vi "Get configuration chain.vi"(8 "error in (no error)":errorcluster, 11 "TemplateBase in":refnum<class "Cobolt.lvclass">) -> (0 "error out":errorcluster, 1 "class name":string[](array[string]), 2 "configuration chain":variant[](array[variant]), 3 "TemplateBase out":refnum<class "Cobolt.lvclass">)   [LabVIEW 2012, in "Cobolt.lvclass"]
doc: "Returns an array of variants containing the configuration clusters of each class in the inheritance chain (lowest child class first), together with an array of all class names in the inheritance chain.\n\nFor classes without configuration cluster, the configuration chain contains empty variants."
uses:
  Cobolt.lvclass
  <vilib>/Distrio/Murmex/Murmex/Murmex.lvclass
  Cobolt.lvclass/Cobolt.ctl
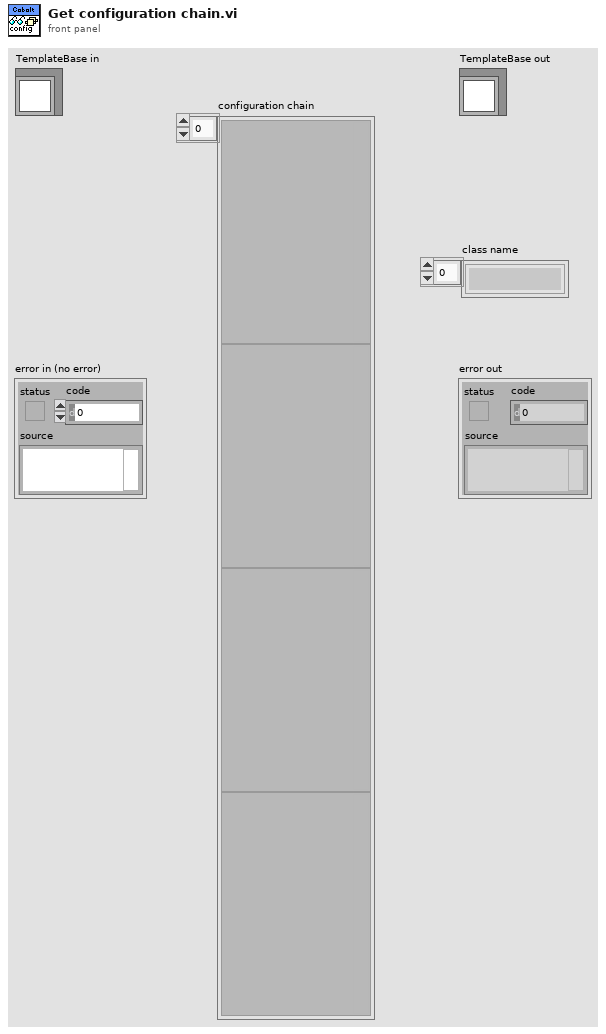
[diagram p1: front panel]
types:
  T1 = typedef "Cobolt.lvclass/configuration_cluster.ctl" = cluster{"VISA resource name":string, "Enable Termination Char":u16, "Baud rate":u32, "data bits":u16, "Flow control":u16, "stop bits":u16, "parity":u16, "Time out":u32, "VISA Wait":dbl[unit], "Laser line":T2, "Generate Error if Fail":bool}
  T2 = typedef "Cobolt.lvclass/laser lines.ctl" = u16
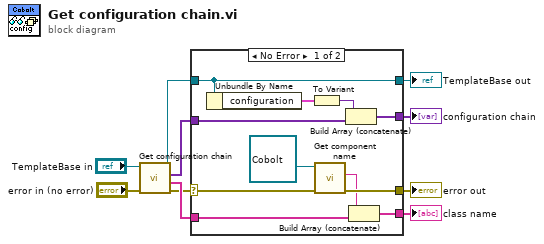
[diagram p0: block diagram]
diagram:
  n1 = call-parent "Get configuration chain.vi"("error in (no error)"="error in (no error)", "MurmexBase in"="TemplateBase in") -> ("error out"=w4:errorcluster, "class name"=w5:string[], "configuration chain"=w7:variant[], "MurmexBase out"=w2:refnum<class "Cobolt.lvclass">)  [unwired: 6 in]
  n2 = case shown="No Error" w4 {
    selector: w4 -> [w18 w25]
    tunnel: [w17 w25] -> w3
    tunnel: [w14 w24] -> w1
    tunnel: w2 -> [w14 w24]
    tunnel: [w19 w22] -> w6
    tunnel: [w15 w23] -> w8
    tunnel: w7 -> [w13 w22]
    tunnel: w5 -> [w12 w23]
    frame No Error {
      n3 = Unbundle By Name(w14) -> ("configuration"=w21:T1)
      n4 = To Variant(anything=w21) -> (Variant=w20:variant)
      n5 = call <vilib>:"Get component name.vi"("error in (no error)"=w18, "Murmex in"=refnum<class "Cobolt.lvclass"> refnum ("Template.lvclass")) -> ("error out"=w17:errorcluster, "component name"=w16:string)  [unwired: 7 in, 1 out]
      n6 = Build Array (concatenate)(w20, w13) -> (w19:variant[])
      n7 = Build Array (concatenate)(w16, w12) -> (w15:string[])
    }
    frame Error {
    }
  }
  "error out" <- w3
  "TemplateBase out" <- w1
  "configuration chain" <- w6
  "class name" <- w8
